vi "S2C_Shared_Proc_ResultGlobal.vi"(7 "Action":enum16{"Init", "Add", "Get"}(ring), 8 "Error In":errorcluster, 11 "Data In":T2) -> (0 "Error Out":errorcluster, 3 "Data Out":T1(array[cluster]))   [LabVIEW 2015]
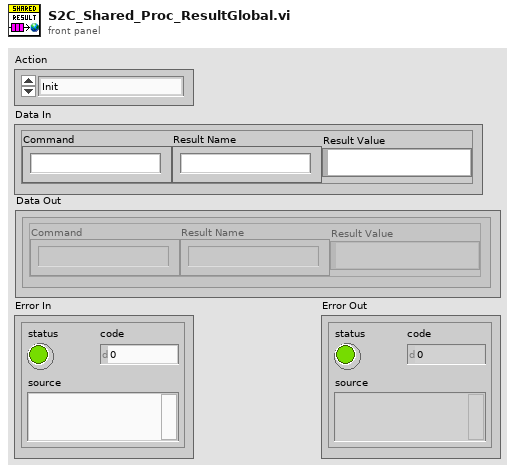
[diagram p1: front panel]
types:
  T1 = cluster{"Command":string, "Result Name":string, "Result Value":variant}[]
  T2 = cluster{"Command":string, "Result Name":string, "Result Value":variant}
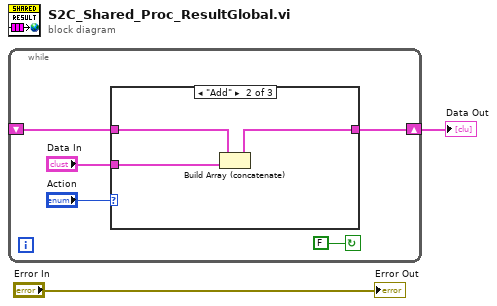
[diagram p0: block diagram]
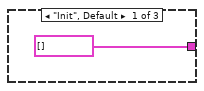
[diagram p2: hidden frame]
diagram:
  n1 = while {
    shift-right: [w5] -> w1
    shift-left: _ -> [w4]
    stop <- FALSE continue-if-true
    n2 = case shown="\"Add\"" "Action" {
      tunnel: [T1 [] ("StepData") w9 w12] -> w5
      tunnel: w4 -> [_ w11 w12]
      tunnel: "Data In" -> [_ w10 _]
      frame "Init", Default {
      }
      frame "Add" {
        n3 = Build Array (concatenate)(w11, w10) -> (w9:T1)
      }
      frame "Get" {
      }
    }
  }
  "Data Out" <- w1
  "Error Out" <- "Error In"
